vi "Deduct_Amount.vi"(0 "Total_Cash_Count_In":T1, 5 "Total_Inserted_Amount":i32) -> (4 "Total_Cash_Count_Out":T1)   [LabVIEW 2021]
doc: "Used to deduct the amount inserted."
uses:
  Controls/Total_Cash_Count.ctl
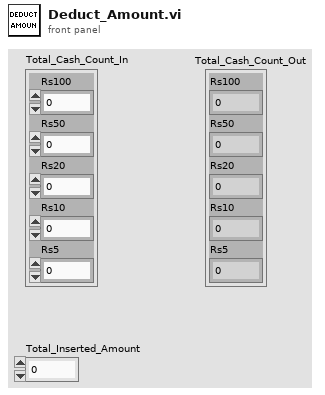
[diagram p1: front panel]
types:
  T1 = typedef "Total_Cash_Count.ctl" = cluster{"Rs100":i32, "Rs50":i32, "Rs20":i32, "Rs10":i32, "Rs5":i32}
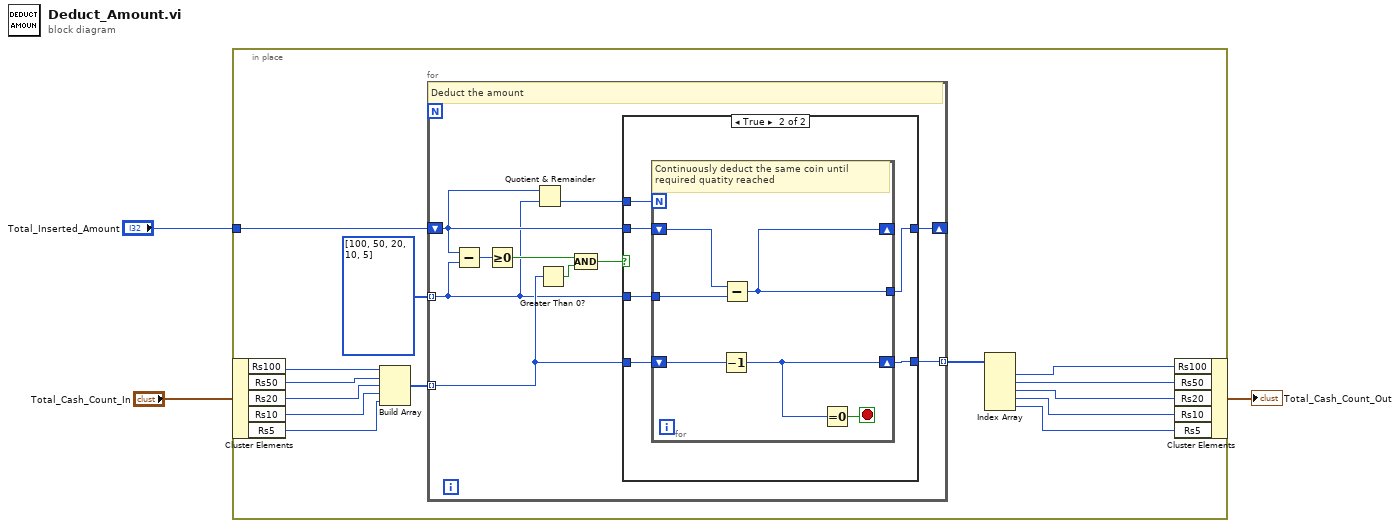
[diagram p0: block diagram]
diagram:
  n1 = in-place {
    in-place-border: "Total_Inserted_Amount" -> [w17]
    n2 = in-place-cluster #1("Total_Cash_Count_In") -> ("Rs100"=w14:i32, "Rs50"=w13:i32, "Rs20"=w12:i32, "Rs10"=w11:i32, "Rs5"=w10:i32)
    n3 = Build Array(w14, w13, w12, w11, w10) -> (w15:i32[])
    n4 = for {
      tunnel: w15 -> [w23] mode=indexing
      shift-right: [w27] -> _
      shift-left: w17 -> [w20]
      tunnel: [w26] -> w9 mode=indexing
      tunnel: i32[] [100, 50, 20, 10, 5] -> [w19] mode=indexing
      # "Deduct the amount"
      n5 = Subtract(x=w20, y=w19) -> (x-y=w25:i32)
      n6 = Greater Or Equal To 0?(x=w25) -> (x >= 0?=w24:bool)
      n7 = Quotient & Remainder(x=w20, y=w19) -> (floor(x/y)=w18:i32)  [unwired: 1 out]
      n8 = Greater Than 0?(x=w23) -> (x > 0?=w21:bool)
      n9 = Compound Arithmetic op=AND(w24, w21) -> (w22:bool)
      n10 = case shown="True" w22 {
        tunnel: w20 -> [w28 w35]
        tunnel: w23 -> [w29 w34]
        tunnel: [w28 w31] -> w27
        tunnel: [w29 w30] -> w26
        tunnel: w19 -> [_ w33]
        tunnel: w18 -> [_ w32]
        frame False {
        }
        frame True {
          n11 = for {
            N: w32 -> [_]
            tunnel: w33 -> [w40]
            shift-right: [w36] -> w30
            shift-left: w34 -> [w37]
            shift-right: [w39] -> _
            shift-left: w35 -> [w41]
            tunnel: [w39] -> w31
            stop <- w38 stop-if-true
            # "Continuously deduct the same coin until required quatity reached"
            n12 = Decrement(x=w37) -> (x-1=w36:i32)
            n13 = Subtract(x=w41, y=w40) -> (x-y=w39:i32)
            n14 = Equal To 0?(x=w36) -> (x = 0?=w38:bool)
          }
        }
      }
    }
    n15 = Index Array(array=w9) -> (element #1=w8:i32, element #2=w7:i32, element #3=w6:i32, element #4=w5:i32, element #5=w4:i32)  [unwired: 5 in]
    n16 = in-place-cluster #1("Rs100"=w8, "Rs50"=w7, "Rs20"=w6, "Rs10"=w5, "Rs5"=w4) -> (→"Total_Cash_Count_Out":T1)
  }
